vi "Download VI Package.vi"(7 "Version":string caption="Version (latest)", 8 "error in (no error)":errorcluster, 9 "File Path":path, 10 "Package Name":string, 11 "Artifactory.VIPM":refnum<class "Artifactory.VIPM.lvclass">) -> (0 "error out":errorcluster, 1 "File Path out":path, 3 "Artifactory.VIPM out":refnum<class "Artifactory.VIPM.lvclass">)   [LabVIEW 2021, in "Artifactory.VIPM.lvclass"]
uses:
  Artifactory.VIPM.lvclass
  C:/Repositories/LVOS/Artifactory/lv-src/Artifactory/Artifactory.lvclass
  <vilib>/Utility/error.llb/Error Cluster From Error Code.vi
  <vilib>/ErrorRing/Error Ring.xnode
  Artifactory/Artifactory.lvclass
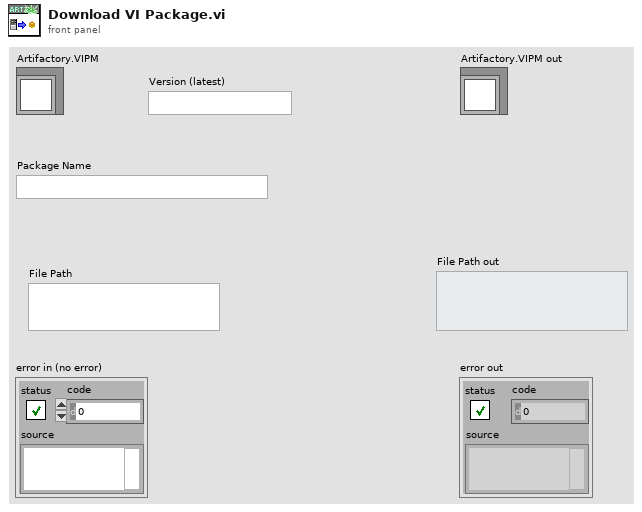
[diagram p1: front panel]
types:
  T1 = cluster{"Major":u8, "Minor":u8, "Fix":u8, "Build":u16}[]
  T2 = cluster{"Major":u8, "Minor":u8, "Fix":u8, "Build":u16}
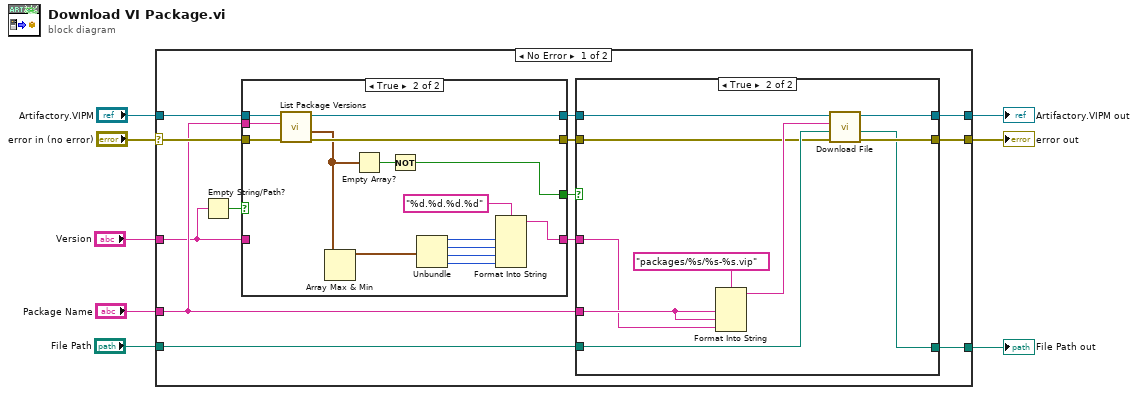
[diagram p0: block diagram]
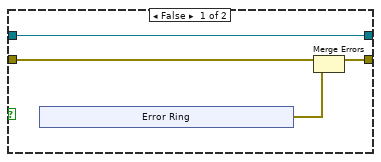
[diagram p2: hidden frame]
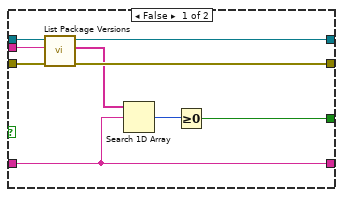
[diagram p3: hidden frame]
diagram:
  n1 = case shown="No Error" "error in (no error)" {
    selector: "error in (no error)" -> [w17 w65]
    tunnel: [w20 w65] -> w7
    tunnel: [w21 w64] -> w5
    tunnel: "Artifactory.VIPM" -> [w14 w64]
    tunnel: "Package Name" -> [w12 _]
    tunnel: "File Path" -> [w18 _]
    tunnel: [w19 _] -> w2
    tunnel: "Version" -> [w11 _]
    frame No Error {
      n2 = Empty String/Path?(string/path=w11) -> (empty?=w13:bool)
      n3 = case shown="True" w13 {
        tunnel: w17 -> [w45 w63]
        tunnel: [w46 w62] -> w16
        tunnel: [w48 w61] -> w15
        tunnel: w14 -> [w47 w60]
        tunnel: w12 -> [w44 w59]
        tunnel: w11 -> [w42 _]
        tunnel: [w42 w52] -> w10
        tunnel: [w40 w49] -> w9
        frame False {
          n4 = call "List Package Versions.vi"("error in (no error)"=w45, "Package Name"=w44, "Artifactory.VIPM in"=w47) -> ("error out"=w46:errorcluster, "Package Versions"=w43:string[], "Artifactory.VIPM out"=w48:refnum<class "Artifactory.VIPM.lvclass">)  [unwired: 5 in, 1 out]
          n5 = Search 1D Array(1D array=w43, element=w42) -> (index of element=w41:i32)  [unwired: 1 in]
          n6 = Greater Or Equal To 0?(x=w41) -> (x >= 0?=w40:bool)
        }
        frame True {
          n7 = call "List Package Versions.vi"("error in (no error)"=w63, "Package Name"=w59, "Artifactory.VIPM in"=w60) -> ("error out"=w62:errorcluster, "Semantic Versions"=w51:T1, "Artifactory.VIPM out"=w61:refnum<class "Artifactory.VIPM.lvclass">)  [unwired: 5 in, 1 out]
          n8 = Array Max & Min(array=w51) -> (max value=w58:T2)  [unwired: 3 out]
          n9 = Empty Array?(array=w51) -> (empty?=w50:bool)
          n10 = Not(x=w50) -> (.not. x?=w49:bool)
          n11 = Unbundle(w58) -> ("Major"=w57:u8, "Minor"=w54:u8, "Fix"=w55:u8, "Build"=w56:u16)
          n12 = Format Into String(format string="%d.%d.%d.%d", w57, w54, w55, w56) -> (resulting string=w52:string)  [unwired: 2 in, 1 out]
        }
      }
      n13 = case shown="True" w9 {
        tunnel: [w25 w39] -> w21
        tunnel: [w23 w38] -> w20
        tunnel: [_ w37] -> w19
        tunnel: w18 -> [_ w34]
        tunnel: w16 -> [w24 w33]
        tunnel: w15 -> [w25 w32]
        tunnel: w12 -> [_ w31]
        tunnel: w10 -> [_ w30]
        frame False {
          n14 = xnode "Error Ring"() -> ("error out"=w22:errorcluster)
          n15 = Merge Errors(w24, w22) -> (w23:errorcluster)
        }
        frame True {
          n16 = Format Into String(format string="packages/%s/%s-%s.vip", w31, w31, w30) -> (resulting string=w35:string)  [unwired: 2 in, 1 out]
          n17 = call "Download File.vi"("error in (no error)"=w33, "File Path"=w34, "Repository Path"=w35, "Artifactory in"=w32) -> ("error out"=w38:errorcluster, "File Path out"=w37:path, "Artifactory out"=w39:refnum<class "Artifactory.VIPM.lvclass">)  [unwired: 5 in]
        }
      }
    }
    frame Error {
    }
  }
  "error out" <- w7
  "Artifactory.VIPM out" <- w5
  "File Path out" <- w2
